vi "OCT Bscan Test.vi"() -> ()   [LabVIEW 2017]
panel:
  out "Intensity Graph":dbl[][](graph)
  in  "Data Range":T1={"Z start (pxl)"=1, "Z length (pxl)"=400}
  in  "# Cscan":i32
  in  "Save Path":path=path "E:/Jiarui/0212test"
  out "error out":errorcluster
  in  "Objective":u16(ring)=1 items=["5X LKM05", "10X LKM10", "20X LKM20", "10X LSM02"]
  in  "ROI Parameters":T2={"ROI (mm)"={"X (mm)"=1.0, "Y (mm)"=1.0}, "Shift (mm)"={"Xshift (mm)"=0.0, "Yshift (mm)"=0.0}}
  in  "Scan Parameters":T3={"# Scan"={"#Ascan"=400, "#Bscan"=400}, "# Rpt"={"#ARpt"=1, "#BRpt"=1}, "Aline Rate"=2, "# Extra"={"# ARpt_extra"=5, "#Brtn_extra"=80}} {"Aline Rate" items=["76 KHz", "146 KHz", "76 KHz", "28 KHz", "10 KHz"]}
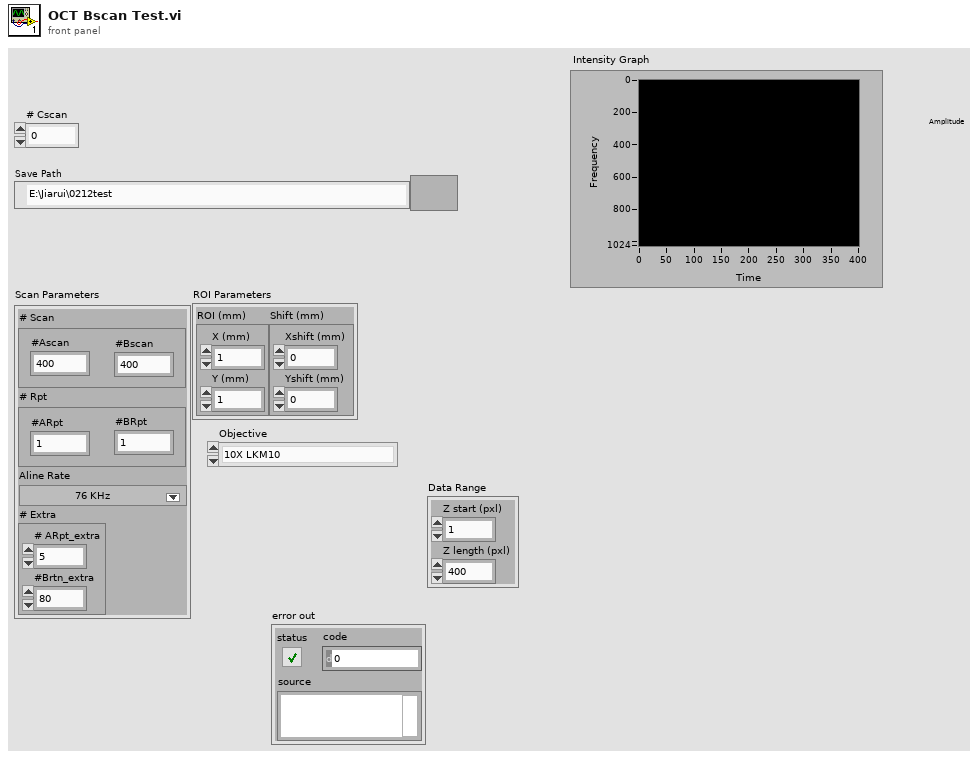
[diagram p1: front panel]
types:
  T1 = cluster{"Z start (pxl)":i32, "Z length (pxl)":i32}
  T2 = cluster{"ROI (mm)":cluster{"X (mm)":dbl, "Y (mm)":dbl}, "Shift (mm)":cluster{"Xshift (mm)":sgl, "Yshift (mm)":sgl}}
  T3 = cluster{"# Scan":cluster{"#Ascan":i32, "#Bscan":i32}, "# Rpt":cluster{"#ARpt":i32, "#BRpt":i32}, "Aline Rate":u16, "# Extra":cluster{"# ARpt_extra":i32, "#Brtn_extra":i32}}
  T4 = enum16{"Init", "Configure", "Configure Data", "Generate Scan Pattern", "Start Acquire Raw", "Start Acquire Data", "Acquire RAW", "Acquire Data", "Stop Acquire", "Uninit"}
  T5 = enum16{"Create", "Enqueue", "Dequeue", "Release"}
  T6 = cluster{"Image Index":i16, "Slice Index":i16, "#Cscan":i32, "nAT per B":i32, "nA per B":i32, "Brtn_extra/2":i32}
  T7 = cluster{"Objective":u16, "Aline Rate":u16, "# Cscan":i32, "ROI Parameters":cluster{"ROI (mm)":cluster{"X (mm)":sgl, "Y (mm)":sgl}, "Shift (mm)":cluster{"Xshift (mm)":sgl, "Yshift (mm)":sgl}}}
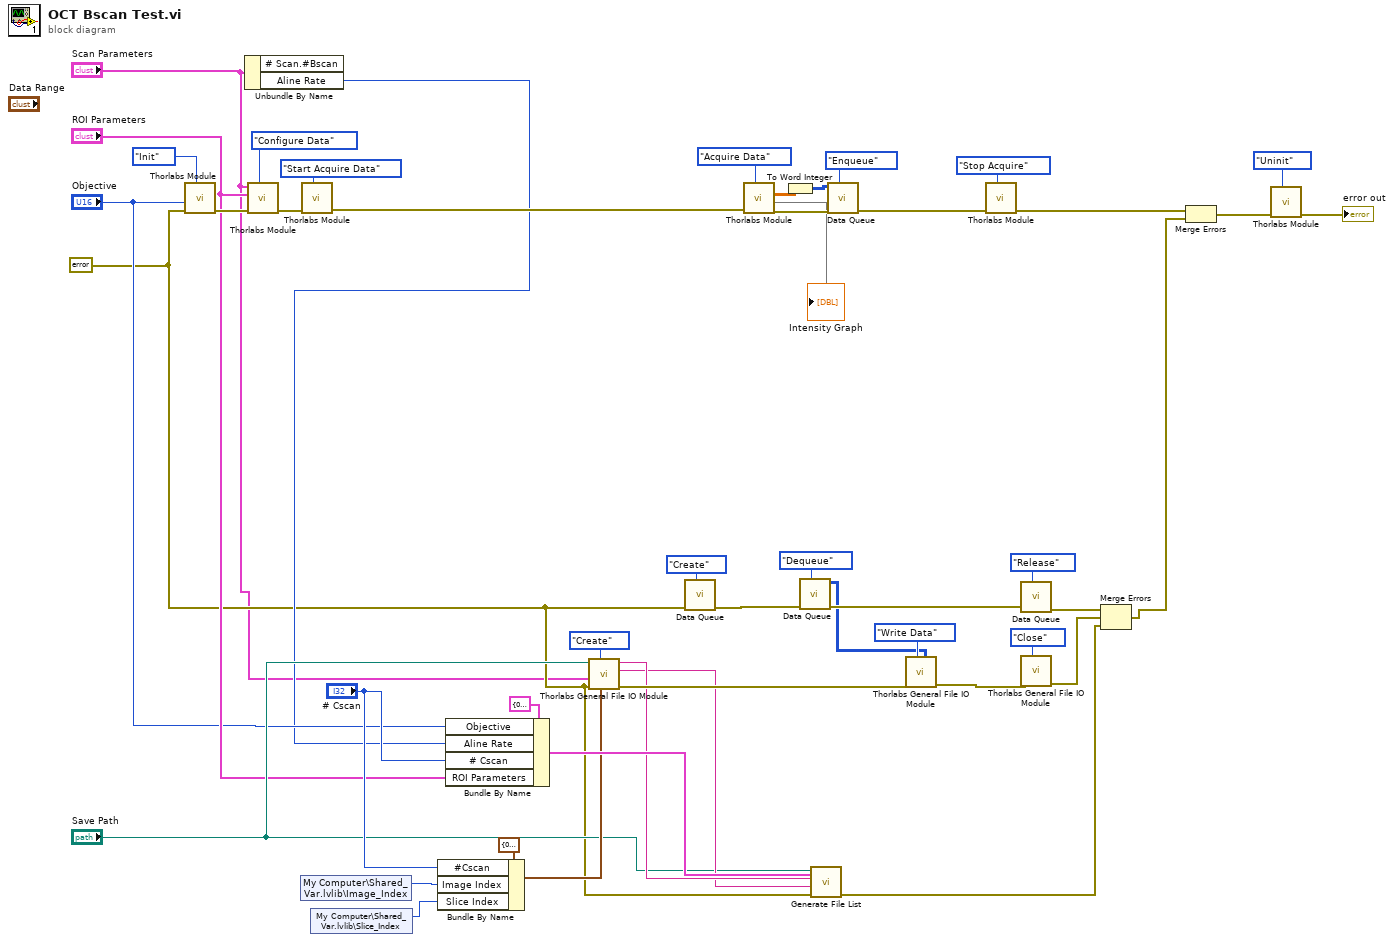
[diagram p0: block diagram]
diagram:
  w7 = errorcluster {"status"=FALSE, "code"=0, "source"=""} ("error in")
  n1 = call "Thorlabs Module.vi"("Actions"=T4."Init", "error in"=w7, "Objective"="Objective") -> ("error out"=w48:errorcluster)  [unwired: 6 in, 2 out]
  n2 = Unbundle By Name("Scan Parameters") -> ("Aline Rate"=w14:u16)  [unwired: 1 out]
  n3 = call "Thorlabs Module.vi"("Actions"=T4."Configure Data", "error in"=w48, "ROI Parameters"="ROI Parameters", "Scan Parameters"="Scan Parameters") -> ("error out"=w47:errorcluster)  [unwired: 5 in, 2 out]
  n4 = shared-variable "My Computer\\Shared_Var.lvlib\\Image_Index"() -> (w23:i16)  [unwired: 1 in, 1 out]
  n5 = call "Thorlabs Module.vi"("Actions"=T4."Start Acquire Data", "error in"=w47) -> ("error out"=w46:errorcluster)  [unwired: 7 in, 2 out]
  n6 = shared-variable "My Computer\\Shared_Var.lvlib\\Slice_Index"() -> (w22:i16)  [unwired: 1 in, 1 out]
  n7 = Bundle By Name(cluster=T6 {"Image Index"=0, "Slice Index"=0, "#Cscan"=0, "nAT per B"=0, "nA per B"=0, "Brtn_extra/2"=0} ("Imaging Parameters"), "#Cscan"="# Cscan", "Image Index"=w23, "Slice Index"=w22) -> (w21:T6)
  n8 = Bundle By Name(cluster=T7 {"Objective"=0, "Aline Rate"=2, "# Cscan"=1, "ROI Parameters"={"ROI (mm)"={"X (mm)"=1.0, "Y (mm)"=1.0}, "Shift (mm)"={"Xshift (mm)"=0.0, "Yshift (mm)"=0.0}}} ("Log Header Parameters"), "Objective"="Objective", "Aline Rate"=w14, "# Cscan"="# Cscan", "ROI Parameters"="ROI Parameters") -> (w28:T7)
  n9 = call "Thorlabs General File IO Module.vi"("Imaging Parameters"=w21, "Actions"=enum16{"Create", "Write", "Write Data", "Close"}."Create", "error in"=w7, "Scan Parameters"="Scan Parameters", "Save Path"="Save Path") -> ("error out"=w32:errorcluster, "Scan Parameter"=w26:string, "Save Name"=w27:string)  [unwired: 4 in]
  n10 = call "Data Queue.vi"("Action"=T5."Create", "error in (no error)"=w7) -> ("error out"=w33:errorcluster)  [unwired: 8 in, 1 out]
  n11 = call "Thorlabs Module.vi"("Actions"=T4."Acquire Data", "error in"=w46) -> ("error out"=w13:errorcluster, "Data Out"=w2:sgl[][], 4:→"Intensity Graph")  [unwired: 6 in, 1 out]
  n12 = To Word Integer(number=w2) -> (16bit integer=w4:i16[][])
  n13 = call "Data Queue.vi"("Action"=T5."Dequeue", "error in (no error)"=w33) -> ("error out"=w35:errorcluster, "Data Out"=w3:u16[][])  [unwired: 8 in]
  n14 = call "Generate File List.vi"(7:w28, "error in (no error)"=w7, 9:w26, "Save Name"=w27, "Save Path"="Save Path") -> ("error out"=w25:errorcluster)  [unwired: 6 in]
  n15 = call "Data Queue.vi"("Action"=T5."Enqueue", "error in (no error)"=w13, "Data In"=w4) -> ("error out"=w42:errorcluster)  [unwired: 7 in, 1 out]
  n16 = call "Thorlabs General File IO Module.vi"("Data In"=w3, "Actions"=enum16{"Create", "Write", "Write Data", "Close"}."Write Data", "error in"=w32) -> ("error out"=w31:errorcluster)  [unwired: 6 in, 2 out]
  n17 = call "Thorlabs Module.vi"("Actions"=T4."Stop Acquire", "error in"=w42) -> ("error out"=w45:errorcluster)  [unwired: 7 in, 2 out]
  n18 = call "Data Queue.vi"("Action"=T5."Release", "error in (no error)"=w35) -> ("error out"=w37:errorcluster)  [unwired: 8 in, 1 out]
  n19 = call "Thorlabs General File IO Module.vi"("Actions"=enum16{"Create", "Write", "Write Data", "Close"}."Close", "error in"=w31) -> ("error out"=w30:errorcluster)  [unwired: 7 in, 2 out]
  n20 = Merge Errors(w37, w30, w25) -> (w10:errorcluster)
  n21 = Merge Errors(w45, w10) -> (w44:errorcluster)
  n22 = call "Thorlabs Module.vi"("Actions"=T4."Uninit", "error in"=w44) -> ("error out"=→"error out":errorcluster)  [unwired: 7 in, 2 out]
